vi "RequestSync.vi"(8 "error in (no error)":errorcluster, 10 "Image Data":string, 11 "InferenceTCP in":refnum<class "InferenceTCP.lvclass">) -> (0 "error out":errorcluster, 2 "Result":bool, 3 "InferenceTCP out":refnum<class "InferenceTCP.lvclass">)   [LabVIEW 2019, in "InferenceTCP.lvlib" / "InferenceTCP.lvclass"]
uses:
  InferenceTCP.lvclass
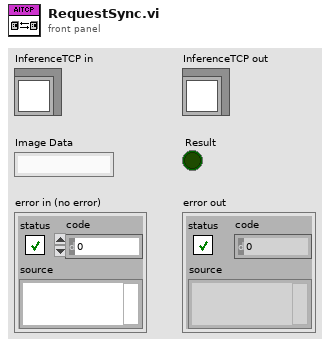
[diagram p1: front panel]
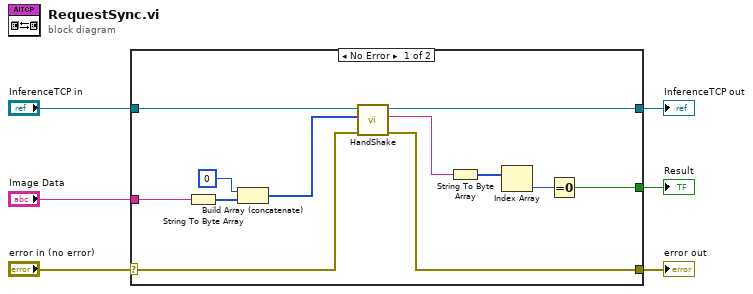
[diagram p0: block diagram]
diagram:
  n1 = case shown="No Error" "error in (no error)" {
    selector: "error in (no error)" -> [w12 w20]
    tunnel: [w11 w20] -> w5
    tunnel: [w13 w19] -> w3
    tunnel: "InferenceTCP in" -> [w14 w19]
    tunnel: "Image Data" -> [w16 _]
    tunnel: [w7 _] -> w1
    frame No Error {
      n2 = String To Byte Array(string=w16) -> (unsigned byte array=w18:u8[])
      n3 = Build Array (concatenate)(u8 0 ("Numeric"), w18) -> (w15:u8[])
      n4 = call "HandShake.vi"("error in (no error)"=w12, "Data In"=w15, "InferenceTCP in"=w14) -> ("error out"=w11:errorcluster, "Data Out"=w10:string, "InferenceTCP out"=w13:refnum<class "InferenceTCP.lvclass">)  [unwired: 6 in]
      n5 = String To Byte Array(string=w10) -> (unsigned byte array=w9:u8[])
      n6 = Index Array(array=w9) -> (element=w8:u8)  [unwired: 1 in]
      n7 = Equal To 0?(x=w8) -> (x = 0?=w7:bool)
    }
    frame Error {
    }
  }
  "error out" <- w5
  "InferenceTCP out" <- w3
  "Result" <- w1
